vi "Msg - Queue Manager Mode.vi"(0 "Mode":T1, 5 "Module Name":string, 11 "error in (no error)":errorcluster) -> (4 ">>ThisModule":refnum<queue>, 6 ">>Controller":refnum<queue>, 15 "error out":errorcluster)   [LabVIEW 2020, in "Template.lvlib"]
doc: "Template used to create VIs that belong to this Module."
uses:
  Template.lvlib
  Controls/Message - Queue Manager Mode.ctl
  Controls/Module - Data.ctl
  Modules.ctl
  Controls/Module - States.ctl
  Controls/Timing - Data.ctl
  Controls/Process - Element.ctl
  Controls/Process.ctl
  Controls/Process - Status.ctl
  Controls/Message.ctl
  Error Handler - Logger Module/Error Handler - Logger.lvlib
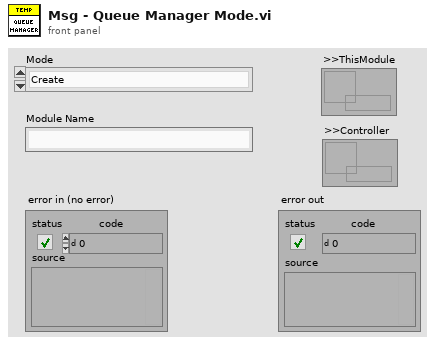
[diagram p1: front panel]
types:
  T1 = typedef "Template.lvlib/Message - Queue Manager Mode.ctl" = enum16{"Create", "Get", "Destroy"}
  T2 = typedef "Template.lvlib/Module - Data.ctl" = cluster{"This Module":T3, "Current State":T4, "Timing Data":T5, "Processes":T6[], "Log":string}
  T3 = typedef "Error Handler - Logger.lvlib/Modules.ctl" = enum16{"Controller", "Error Handler - Logger"}
  T4 = typedef "Template.lvlib/Module - States.ctl" = enum16{"Initialize", "Event ", "Send data", "FP Element: Update", "FP Element: Disable/Enable", "Timer: Setup", "Terminate", "---------------Template---------------"}
  T5 = typedef "Template.lvlib/Timing - Data.ctl" = cluster{"Elapsed Time":dbl, "Time Target":dbl, "Time Stamp":timestamp, "Paused?":bool, "Reached?":bool}
  T6 = typedef "Template.lvlib/Process - Element.ctl" = cluster{"Process":T7, "Status":T8, "Data":variant}
  T7 = typedef "Template.lvlib/Process.ctl" = enum16{""}
  T8 = typedef "Template.lvlib/Process - Status.ctl" = enum16{"Uninitialized", "Busy"}
  T9 = typedef "Template.lvlib/Message.ctl" = cluster{"State":T4, "Data":variant, "Transitioning State?":bool}
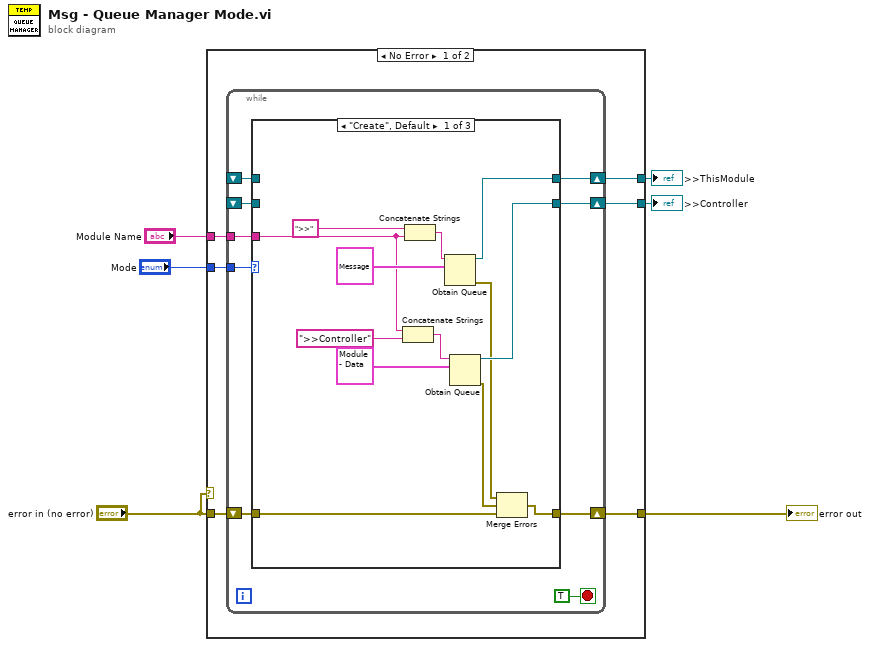
[diagram p0: block diagram]
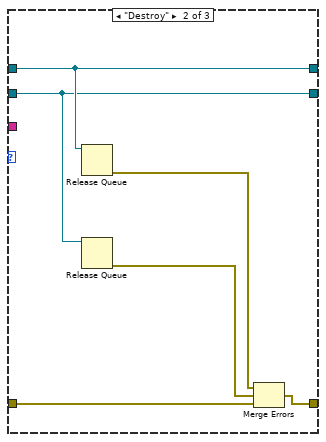
[diagram p2: hidden frame]
diagram:
  n1 = case shown="No Error" "error in (no error)" {
    tunnel: [w12 _] -> w1
    tunnel: [w11 w44] -> w6
    tunnel: "error in (no error)" -> [w10 w44]
    tunnel: [w9 _] -> w3
    tunnel: "Mode" -> [w8 _]
    tunnel: "Module Name" -> [w7 _]
    frame No Error {
      n2 = while {
        shift-right: [w21] -> w12
        shift-left: _ -> [w20]
        shift-right: [w19] -> w11
        shift-left: w10 -> [w18]
        shift-right: [w15] -> w9
        shift-left: _ -> [w16]
        tunnel: w8 -> [w14]
        tunnel: w7 -> [w13]
        stop <- TRUE stop-if-true
        n3 = case shown="\"Create\", Default" w14 {
          tunnel: [w32 w38 w43] -> w21
          tunnel: w20 -> [_ w38 w43]
          tunnel: [w33 w39 w42] -> w19
          tunnel: w18 -> [w34 w40 w42]
          tunnel: [w31 w37 w41] -> w15
          tunnel: w16 -> [_ w37 w41]
          tunnel: w13 -> [w24 _ _]
          frame "Create", Default {
            n4 = Concatenate Strings(w24, ">>Controller" ("name (unnamed)")) -> (w23:string)
            n5 = Concatenate Strings(">>" ("string"), w24) -> (w28:string)
            n6 = Obtain Queue(name (unnamed)=w28, element data type=T9 {"State"=enum."Initialize", "Data"=variant, "Transitioning State?"=FALSE} ("Message")) -> (queue out=w32:refnum<queue>, error out=w26:errorcluster)  [unwired: 3 in, 1 out]
            n7 = Obtain Queue(name (unnamed)=w23, element data type=T2 {"This Module"=enum."Controller", "Current State"=enum."Initialize", "Timing Data"={"Elapsed Time"=0.0, "Time Target"=0.0, "Time Stamp"=timestamp(0 s since 1904-01-01), "Paused?"=FALSE, "Reached?"=FALSE}, "Processes"=[], "Log"=""} ("Module Data")) -> (queue out=w31:refnum<queue>, error out=w22:errorcluster)  [unwired: 3 in, 1 out]
            n8 = Merge Errors(w26, w22, w34) -> (w33:errorcluster)
          }
          frame "Destroy" {
            n9 = Release Queue(queue=w38) -> (error out=w36:errorcluster)  [unwired: 2 in, 2 out]
            n10 = Release Queue(queue=w37) -> (error out=w35:errorcluster)  [unwired: 2 in, 2 out]
            n11 = Merge Errors(w36, w35, w40) -> (w39:errorcluster)
          }
          frame "Get" {
          }
        }
      }
    }
    frame Error {
    }
  }
  "error out" <- w6
  ">>Controller" <- w3
  ">>ThisModule" <- w1
